vi "High Throughput Streaming - Through Memory (Host).vi"() -> ()   [LabVIEW 2016]
doc: "Example Description:\nStreams data through host memory from a RIO device then back to the RIO device at the specified rate(s).\n\nVI Configuration:\nThis example uses the PXI-7966R as the FPGA target by default. To use this VI with another FPGA target, use the following steps to configure the host VI to use a VI configured for your FPGA target:\n\n1. On the block diagram, right-click the Open FPGA VI Reference (PXI-7966R) VI and select Configure Open FPGA VI Reference.\n2. Browse for a new target by clicking the Browse Project button in the Open VI section.\n3. Select the VI under the target that matches your device. Click OK to select this VI.\n4. Click OK to exit the dialog box and to apply the new selection to the FPGA VI.\n\nRunning the VI:\n1. Select a RIO Resource that corresponds to the FPGA device configured above.\n2. Configure the Requested host Buffer Depth, Read/Write Size, and Requested (M) controls on the Host VI Front Panel.\n3. Click the run arrow to run the VI.\n4. Observe the Status of the Host Buffer as well as the Input and Output DMA FIFOs\n5. Observe the achieved Streaming Throughput.\n6. Click Stop on the Front Panel to stop the example\n\n\nExecution Steps:\nRefer to the block diagram of the Host VI for each example to view the execution steps for that specific example."
uses:
  <vilib>/userdefined/High Color/nirio_resource_hc.ctl
  <vilib>/FPGAPlugInAG/PXIe-7966R/niLvFpga_Open_PXIe-7966R.vi
  <vilib>/rvi/interface/common/dynamic/niFpgaDynamicAddResources.vi
  <vilib>/Utility/error.llb/Error Cluster From Error Code.vi
  <vilib>/rvi/errors/niLvFpgaAdjustHostInterfaceError.vi
  <vilib>/FPGAPlugInAG/Dynamic/niLvFpga_Run_Dynamic.vi
  <vilib>/rvi/interface/common/niFpgaWaitOnOcc.vi
  <vilib>/FPGAPlugInAG/Dynamic/niLvFpga_Close_Dynamic.vi
  <vilib>/rvi/interface/nirviOpenFPGA/nirviOpenFPGA.xnode
  FPGA Bitfiles/HighThroug_PXIe-7966R.lvbitx
  <vilib>/rvi/interface/nirviReadWriteControl/nirviReadWriteControl.xnode
  <vilib>/rvi/interface/nirviMethod/nirviMethod.xnode
  <vilib>/rvi/interface/nirviCloseFPGA/nirviCloseFPGA.xnode
  <vilib>/rvi/interface/Simulation/niFpgaSimulationCallBeginRW.vi
  <vilib>/rvi/errors/niLvFpgaMergeErrorWithErrorCode.vi
  <vilib>/FPGAPlugInAG/Dynamic/niLvFpga_ConfigureFifo_Dynamic.vi
  <vilib>/FPGAPlugInAG/Dynamic/niLvFpga_StartFifo_Dynamic.vi
  <vilib>/FPGAPlugInAG/Dynamic/niLvFpga_AcquireReadRegionFifo_Dynamic.vi
  <vilib>/FPGAPlugInAG/Dynamic/niLvFpga_AcquireWriteRegionFifo_Dynamic.vi
  NiFpgaLv.dll
panel:
  out "error out":errorcluster
  in  "Stop":bool
  out "output.Host Buffer Status":cluster{u32, u32, u32}(slide) caption="Host Output Buffer Status" scale=0.0..67108864.0 scale format="%#.1p"
  out "input.Host Buffer Status":cluster{u32, u32, u32}(slide) caption="Host Input Buffer Status" scale=0.0..67108864.0 scale format="%#.1p"
  out "input.Host Buffer Depth (samples)":u32
  out "output.Host Buffer Depth (samples)":u32
  in  "Read/Write Size (samples)":u32=4194304 step=1048576
  in  "Requested Host Buffer Depth (samples)":u32=67108864 step=1048576
  in  "resource name":T1="Select RIO resource"
  out "output.Ever Timed Out?":bool caption="Overflow"
  in  "output.Reset":bool caption="Reset"
  out "output.FPGA FIFO Status":cluster{u32, u32}(slide) caption="FIFO Status" scale=0.0..65559.0 scale format="%#.1p"
  out "output.Max Throughput":u16 caption="Maximum (M)"
  in  "output.Requested Throughput":u16=1000 caption="Requested (M)" step=5
  out "output.Throughput (B/s)":dbl caption="Actual" format="%#.1p"
  out "input.Ever Timed Out?":bool caption="Overflow"
  in  "input.Reset":bool caption="Reset"
  out "input.FPGA FIFO Status":cluster{u32, u32}(slide) caption="FIFO Status" scale=0.0..65535.0 scale format="%#.1p"
  out "input.Max Throughput":u16 caption="Maximum (M)"
  in  "input.Requested Throughput":u16=1000 caption="Requested (M)" step=5
  out "input.Throughput (B/s)":dbl caption="Actual" format="%#.1p"
  out "Stop...":bool
  # "Configuration"
  # "Host"
  # "Input FPGA"
  # "Throughput (B/s)"
  # "Output FPGA"
  # "Throughput (B/s)"
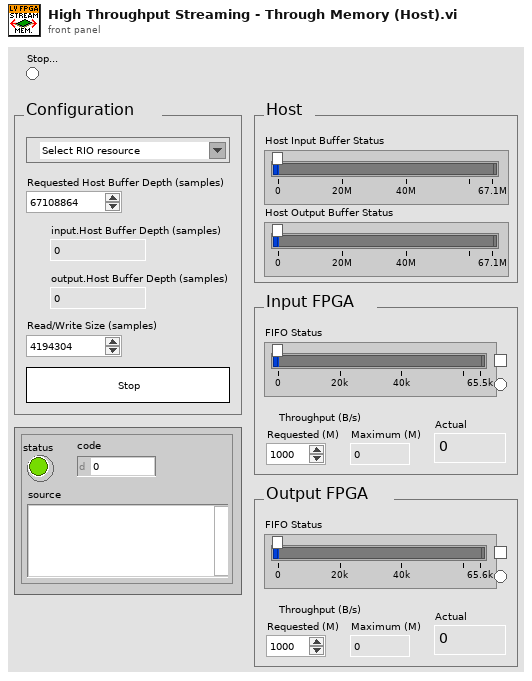
[diagram p1: front panel]
types:
  T1 = typedef "nirio_resource_hc.ctl" = tag
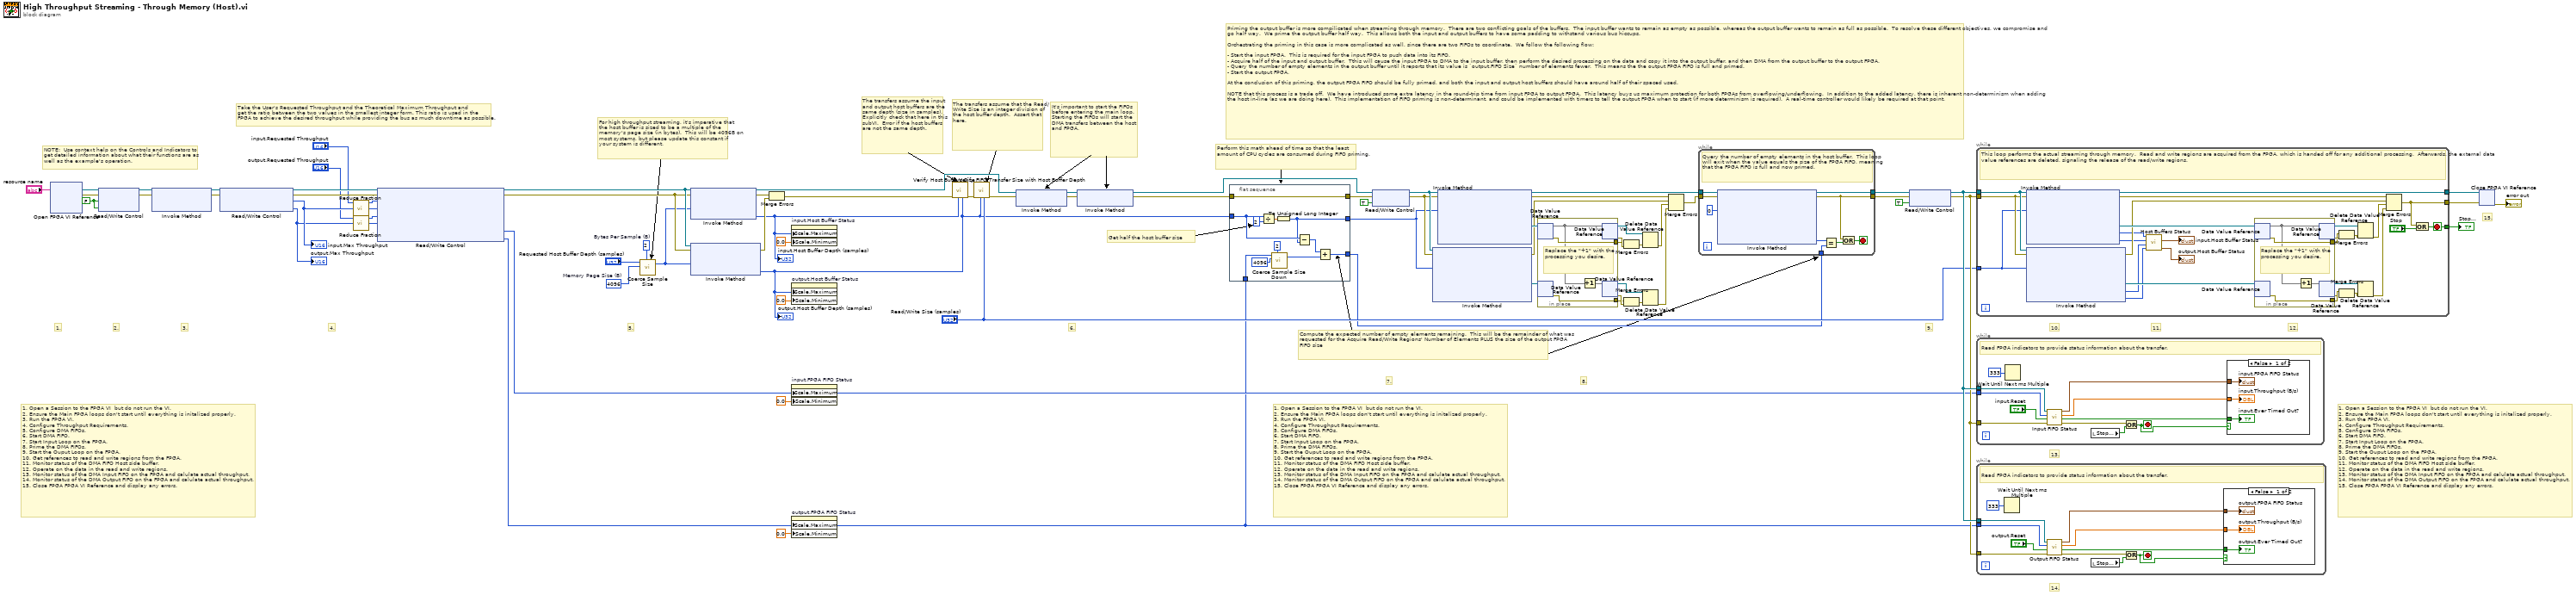
[diagram p0: block diagram]
diagram:
  w60 = u64 4096  # Memory Page Size (B)
  w62 = u64 2  # Bytes Per Sample (B)
  w70 = FALSE ("input.Start")
  # "1. Open a Session to the FPGA VI  but do not run the VI.\n2. Ensure the Main FPGA loops don't start until everything is initalized properly. \n3. Run the FPGA VI.\n4. Configure Throughput Requirements.\n5. Configure DMA FIFOs.\n6. Start DMA FIFO.\n7. Start Input Loop on the FPGA.\n8. Prime the DMA FIFOs.\n9. Start the Ouput Loop on the FPGA.\n10. Get references to read and write regions from the FPGA.\n11. Monitor status of the DMA FIFO Host side buffer.\n12. Operate on the data in the read and write regions. \n13. Monitor status of the DMA Input FIFO on the FPGA and calulate actual throughput.\n14. Monitor status of the DMA Output FIFO on the FPGA and calulate actual throughput.\n15. Close FPGA FPGA VI Reference and display any errors."
  # "1. Open a Session to the FPGA VI  but do not run the VI.\n2. Ensure the Main FPGA loops don't start until everything is initalized properly. \n3. Run the FPGA VI.\n4. Configure Throughput Requirements.\n5. Configure DMA FIFOs.\n6. Start DMA FIFO.\n7. Start Input Loop on the FPGA.\n8. Prime the DMA FIFOs.\n9. Start the Ouput Loop on the FPGA.\n10. Get references to read and write regions from the FPGA.\n11. Monitor status of the DMA FIFO Host side buffer.\n12. Operate on the data in the read and write regions. \n13. Monitor status of the DMA Input FIFO on the FPGA and calulate actual throughput.\n14. Monitor status of the DMA Output FIFO on the FPGA and calulate actual throughput.\n15. Close FPGA FPGA VI Reference and display any errors."
  # "12."
  # "10."
  # "15."
  # "Take the User's Requested Throughput and the Theoretical Maximum Throughput and\nget the ratio between the two values in the smallest integer form. This ratio is used in the \nFPGA to achieve the desired throughput while providing the bus as much downtime as possible."
  # "9."
  # "11."
  # "14."
  # "13."
  # "8."
  # "7."
  # "6."
  # "5."
  # "4."
  # "3."
  # "2."
  # "1. Open a Session to the FPGA VI  but do not run the VI.\n2. Ensure the Main FPGA loops don't start until everything is initalized properly. \n3. Run the FPGA VI.\n4. Configure Throughput Requirements.\n5. Configure DMA FIFOs.\n6. Start DMA FIFO.\n7. Start Input Loop on the FPGA.\n8. Prime the DMA FIFOs.\n9. Start the Ouput Loop on the FPGA.\n10. Get references to read and write regions from the FPGA.\n11. Monitor status of the DMA FIFO Host side buffer.\n12. Operate on the data in the read and write regions. \n13. Monitor status of the DMA Input FIFO on the FPGA and calulate actual throughput.\n14. Monitor status of the DMA Output FIFO on the FPGA and calulate actual throughput.\n15. Close FPGA FPGA VI Reference and display any errors."
  # "1."
  # "NOTE:  Use context help on the Controls and Indicators to \nget detailed information about what their functions are as\nwell as the example's operation."
  # "Compute the expected number of empty elements remaining.  This will be the remainder of what was requested for the Acquire Read/Write Regions' Number of Elements PLUS the size of the output FPGA FIFO size"
  # "Get half the host buffer size"
  # "Perform this math ahead of time so that the least amount of CPU cycles are consumed during FIFO priming."
  # "Priming the output buffer is more compilicated when streaming through memory.  There are two conflicting goals of the buffers.  The input buffer wants to remain as empty as possible, whereas the output buffer wants to remain as full as possible.  To resolve these different objectives, we compromise and go half way.  We prime the output buffer half way.  This allows both the input and output buffers to have some padding to withstand various bus hiccups.\n\nOrchestrating the priming in this case is more complicated as well, since there are two FIFOs to coordinate.  We follow the following flow:\n\n- Start the input FPGA.  This is required for the input FPGA to push data into its FIFO.\n- Acquire half of the input and output buffer.  Tthis will cause the input FPGA to DMA to the input buffer, then perform the desired processing on the data and copy it into the output buffer, and then DMA from the output buffer to the output FPGA.\n- Query the number of empty elements in the output buffer until it reports that its value is `output.FIFO Size` number of elements fewer.  This means the the output FPGA FIFO is full and primed.\n- Start the output FPGA.\n\nAt the conclusion of this priming, the output FPGA FIFO should be fully primed, and both the input and output host buffers should have around half of their spaced used.\n\nNOTE that this process is a trade off.  We have introduced some extra latency in the round-trip time from input FPGA to output FPGA.  This latency buys us maximum protection for both FPGAs from overflowing/underflowing.  In addition to the added latency, there is inherent non-determinism when adding the host in-line (as we are doing here).  This implementation of FIFO priming is non-determinant, and could be implemented with timers to tell the output FPGA when to start (if more determinism is required).  A real-time controller would likely be required at that point."
  # "For high throughput streaming, it's imperative that the host buffer is sized to be a multiple of the memory's page size (in bytes).  This will be 4096B on most systems, but please update this constant if your system is different."
  # "It's important to start the FIFOs before entering the main loop.  Starting the FIFOs will start the DMA transfers between the host and FPGA."
  # "The transfers assume that the Read/Write Size is an integer division of the host buffer depth.  Assert that here."
  # "The transfers assume the input and output host buffers are the same depth (size in samples).  Explicitly check that here in this subVI.  Error if the host buffers are not the same depth."
  n1 = xnode "Open FPGA VI Reference"("resource name"="resource name") -> ("FPGA VI Reference Out"=w72:refnum<k20>, "error out"=w71:errorcluster)  [unwired: 1 in]
  n2 = xnode "Read/Write Control"("FPGA VI Reference In"=w72, "error in"=w71, "input.Start"=w70, "output.Start"=w70) -> ("FPGA VI Reference Out"=w65:refnum<k20>, "error out"=w66:errorcluster)
  n3 = xnode "Invoke Method"("FPGA VI Reference In"=w65, "error in"=w66) -> ("FPGA VI Reference Out"=w42:refnum<k20>, "error out"=w41:errorcluster)  [unwired: 1 in]
  n4 = xnode "Read/Write Control"("FPGA VI Reference In"=w42, "error in"=w41) -> ("FPGA VI Reference Out"=w40:refnum<k20>, "error out"=w39:errorcluster, "input.Max Throughput"=w34:u16, "output.Max Throughput"=w33:u16)
  "input.Max Throughput" <- w34
  "output.Max Throughput" <- w33
  n5 = call "Reduce Fraction.vi"("denominator"=w34, "numerator"="input.Requested Throughput") -> ("reduced denominator"=w38:u16, "reduced numerator"=w35:u16)  [unwired: 2 in]
  n6 = call "Reduce Fraction.vi"("denominator"=w33, "numerator"="output.Requested Throughput") -> ("reduced denominator"=w37:u16, "reduced numerator"=w36:u16)  [unwired: 2 in]
  n7 = xnode "Read/Write Control"("FPGA VI Reference In"=w40, "error in"=w39, "input.Requested Throughput"=w35, "input.Requested Throughput Denominator"=w38, "output.Requested Throughput"=w36, "output.Requested Throughput Denominator"=w37) -> ("FPGA VI Reference Out"=w58:refnum<k20>, "error out"=w57:errorcluster, "input.FIFO Size"=w43:u32, "output.FIFO Size"=w8:u32)
  n8 = call "Coerce Sample Size.vi"("Bytes Per Sample (B)"=w62, "Coerce To (B)"=w60, "Size (samples)"="Requested Host Buffer Depth (samples)") -> ("Coerced Size (samples)"=w56:u64)  [unwired: 4 in]
  n9 = xnode "Invoke Method"("FPGA VI Reference In"=w58, "error in"=w57, "Requested Depth"=w56) -> ("FPGA VI Reference Out"=w49:refnum<k20>, "error out"=w54:errorcluster, "Actual Depth"=w1:u32)
  "input.Host Buffer Depth (samples)" <- w1
  n10 = xnode "Invoke Method"("FPGA VI Reference In"=w58, "error in"=w57, "Requested Depth"=w56) -> ("error out"=w53:errorcluster, "Actual Depth"=w2:u32)  [unwired: 1 out]
  "output.Host Buffer Depth (samples)" <- w2
  n11 = Merge Errors(w54, w53) -> (w52:errorcluster)
  n12 = property on="input.Host Buffer Status" class="Slide (strict)"("Scale.Maximum"=w1, "Scale.Minimum"=0.0 ("Scale.Range:Minimum")) -> ()  [unwired: 2 in, 2 out]
  n13 = property on="output.Host Buffer Status" class="Slide (strict)"("Scale.Maximum"=w2, "Scale.Minimum"=0.0 ("Scale.Range:Minimum")) -> ()  [unwired: 2 in, 2 out]
  n14 = property on="input.FPGA FIFO Status" class="Slide (strict)"("Scale.Maximum"=w43, "Scale.Minimum"=0.0 ("Scale.Range:Minimum")) -> ()  [unwired: 2 in, 2 out]
  n15 = property on="output.FPGA FIFO Status" class="Slide (strict)"("Scale.Maximum"=w8, "Scale.Minimum"=0.0 ("Scale.Range:Minimum")) -> ()  [unwired: 2 in, 2 out]
  n16 = call "Verify Host Buffers Size.vi"("output.Host Buffer Size"=w2, "input.Host Buffer Size"=w1, "error in"=w52) -> ("error out"=w51:errorcluster)  [unwired: 8 in]
  n17 = call "Verify FIFO Transfer Size with Host Buffer Depth.vi"("Read/Write Size (samples)"="Read/Write Size (samples)", "Host Buffer Depth (samples)"=w2, "error in"=w51) -> ("error out"=w48:errorcluster)  [unwired: 8 in]
  n18 = xnode "Invoke Method"("FPGA VI Reference In"=w49, "error in"=w48) -> ("FPGA VI Reference Out"=w46:refnum<k20>, "error out"=w47:errorcluster)
  n19 = xnode "Invoke Method"("FPGA VI Reference In"=w46, "error in"=w47) -> ("FPGA VI Reference Out"=w4:refnum<k20>, "error out"=w6:errorcluster)
  n20 = flat-sequence {
    tunnel: w8 -> [w83]
    tunnel: w2 -> [w82]
    tunnel: [w78] -> w7
    tunnel: w6 -> [w77]
    tunnel: [w77] -> w5
    tunnel: [w75] -> w3
    frame #0 {
      n21 = Divide(x=w82, y=u32 2) -> (x/y=w79:dbl)
      n22 = call "Coerce Sample Size Down.vi"("Bytes Per Sample (B)"=u64 2, "Coerce To (B)"=u64 4096, "Size (samples)"=w83) -> ("Coerced Size (samples)"=w80:u64)  [unwired: 4 in]
      n23 = To Unsigned Long Integer(number=w79) -> (unsigned 32bit integer=w78:u32)
      n24 = Subtract(x=w82, y=w78) -> (x-y=w81:u32)
      n25 = Add(x=w81, y=w80) -> (x+y=w75:u64)
    }
  }
  n26 = xnode "Read/Write Control"("FPGA VI Reference In"=w4, "error in"=w5, "input.Start"=TRUE) -> ("FPGA VI Reference Out"=w29:refnum<k20>, "error out"=w28:errorcluster)
  n27 = xnode "Invoke Method"("FPGA VI Reference In"=w29, "error in"=w28, "Number of Elements"=w7) -> ("error out"=w14:errorcluster, "Write Region Reference"=w26:refnum<data-value>)  [unwired: 1 in, 3 out]
  n28 = xnode "Invoke Method"("FPGA VI Reference In"=w29, "error in"=w28, "Number of Elements"=w7) -> ("FPGA VI Reference Out"=w10:refnum<k20>, "error out"=w25:errorcluster, "Read Region Reference"=w27:refnum<data-value>)  [unwired: 1 in, 2 out]
  n29 = in-place {
    in-place-border: [w89] -> w19
    in-place-border: [w88] -> w17
    # "Replace the \"+1\" with the processing you desire."
    # "Insert additional processing here"
    n30 = in-place-dvr #1(w27) -> (w87:i16[], w88:errorcluster)
    n31 = in-place-dvr #2(w26) -> (w89:errorcluster)  [unwired: 1 out]
    n32 = Increment(x=w87) -> (x+1=w86:i16[])
    n33 = in-place-dvr #1(w87) -> (w22:refnum<data-value>, w18:errorcluster)
    n34 = in-place-dvr #2(w86) -> (w21:refnum<data-value>, w20:errorcluster)
  }
  n35 = Merge Errors(w17, w18) -> (w24:errorcluster)
  n36 = Merge Errors(w19, w20) -> (w23:errorcluster)
  n37 = Delete Data Value Reference(data value reference=w22, error in=w24) -> (error out=w15:errorcluster)  [unwired: 1 out]
  n38 = Delete Data Value Reference(data value reference=w21, error in=w23) -> (error out=w16:errorcluster)  [unwired: 1 out]
  n39 = Merge Errors(w25, w14, w15, w16) -> (w9:errorcluster)
  n40 = while {
    tunnel: w9 -> [w98]
    tunnel: [w95] -> w12
    tunnel: w10 -> [w97]
    tunnel: w3 -> [w93]
    tunnel: [w90] -> w11
    stop <- w96 stop-if-true
    # "Query the number of empty elements in the host buffer.  This loop will exit when the value equals the size of the FPGA FIFO, meaning that the FPGA FIFO is full and now primed."
    n41 = xnode "Invoke Method"("FPGA VI Reference In"=w97, "error in"=w98, "Number of Elements"=u32 0) -> ("FPGA VI Reference Out"=w90:refnum<k20>, "error out"=w95:errorcluster, "Empty Elements Remaining"=w91:u32)  [unwired: 1 in, 2 out]
    n42 = Equal?(x=w91, y=w93) -> (x = y?=w94:bool)
    n43 = Or(x=w95, y=w94) -> (x .or. y?=w96:bool)
  }
  n44 = xnode "Read/Write Control"("FPGA VI Reference In"=w11, "error in"=w12, "output.Start"=TRUE ("Start")) -> ("FPGA VI Reference Out"=w64:refnum<k20>, "error out"=w63:errorcluster)
  n45 = while {
    tunnel: w64 -> [w125]
    tunnel: w63 -> [w124]
    tunnel: "Read/Write Size (samples)" -> [w107]
    tunnel: [w119] -> w69
    tunnel: [w118] -> w67
    tunnel: [w116] -> w68
    stop <- w116 stop-if-true
    # "This loop performs the actual streaming through memory.  Read and write regions are acquired from the FPGA, which is handed off for any additional processing.  Afterwards, the external data value references are deleted, signaling the release of the read/write regions."
    n46 = xnode "Invoke Method"("FPGA VI Reference In"=w125, "error in"=w124, "Number of Elements"=w107) -> ("FPGA VI Reference Out"=w119:refnum<k20>, "error out"=w106:errorcluster, "Read Region Reference"=w123:refnum<data-value>, "Elements In Region"=w99:u32, "Elements Remaining"=w102:u32)  [unwired: 1 in]
    n47 = xnode "Invoke Method"("FPGA VI Reference In"=w125, "error in"=w124, "Number of Elements"=w107) -> ("error out"=w105:errorcluster, "Write Region Reference"=w122:refnum<data-value>, "Elements In Region"=w104:u32, "Empty Elements Remaining"=w103:u32)  [unwired: 1 in, 1 out]
    n48 = call "Host Buffers Status.vi"("output.Empty Elements Remaining"=w103, "output.Elements In Region"=w104, "input.Elements Remaining"=w102, "input.Elements In Region"=w99) -> ("output.Host Buffer Status"=→"output.Host Buffer Status":cluster{u32, u32, u32}, "input.Host Buffer Status"=→"input.Host Buffer Status":cluster{u32, u32, u32})  [unwired: 4 in, 2 out]
    n49 = in-place {
      in-place-border: [w129] -> w111
      in-place-border: [w128] -> w108
      # "Replace the \"+1\" with the processing you desire."
      # "Insert additional processing here"
      n50 = in-place-dvr #3(w123) -> (w127:i16[], w128:errorcluster)
      n51 = in-place-dvr #4(w122) -> (w129:errorcluster)  [unwired: 1 out]
      n52 = Increment(x=w127) -> (x+1=w126:i16[])
      n53 = in-place-dvr #3(w127) -> (w115:refnum<data-value>, w109:errorcluster)
      n54 = in-place-dvr #4(w126) -> (w114:refnum<data-value>, w110:errorcluster)
    }
    n55 = Merge Errors(w108, w109) -> (w112:errorcluster)
    n56 = Merge Errors(w111, w110) -> (w113:errorcluster)
    n57 = Delete Data Value Reference(data value reference=w115, error in=w112) -> (error out=w121:errorcluster)  [unwired: 1 out]
    n58 = Delete Data Value Reference(data value reference=w114, error in=w113) -> (error out=w120:errorcluster)  [unwired: 1 out]
    n59 = Merge Errors(w106, w105, w121, w120) -> (w118:errorcluster)
    n60 = Compound Arithmetic op=OR(w118, "Stop") -> (w116:bool)
  }
  "Stop..." <- w68
  n61 = while {
    tunnel: w63 -> [w138]
    tunnel: w43 -> [w136]
    tunnel: w64 -> [w135]
    stop <- w130 stop-if-true
    # "Read FPGA indicators to provide status information about the transfer."
    n62 = Wait Until Next ms Multiple(millisecond multiple=u32 333) -> ()  [unwired: 1 out]
    n63 = call "Input FIFO Status.vi"("error in"=w138, "input.Reset"="input.Reset", "input.FIFO Size"=w136, "FPGA VI Reference"=w135) -> ("error out"=w134:errorcluster, "input.Ever Timed Out?"=w133:bool, "input.Throughput (B/s)"=w132:dbl, "input.FPGA FIFO Status"=w131:cluster{u32, u32})  [unwired: 3 in]
    n64 = local read "Stop..."() -> (w139:bool)
    n65 = Or(x=w134, y=w139) -> (x .or. y?=w130:bool)
    n66 = case shown="False" w130 {
      tunnel: w133 -> [w143 _]
      tunnel: w132 -> [w142 _]
      tunnel: w131 -> [w141 _]
      frame False {
        "input.Throughput (B/s)" <- w142
        "input.Ever Timed Out?" <- w143
        "input.FPGA FIFO Status" <- w141
      }
      frame True {
      }
    }
  }
  n67 = while {
    tunnel: w64 -> [w145]
    tunnel: w63 -> [w153]
    tunnel: w8 -> [w151]
    stop <- w144 stop-if-true
    # "Read FPGA indicators to provide status information about the transfer."
    n68 = Wait Until Next ms Multiple(millisecond multiple=u32 333) -> ()  [unwired: 1 out]
    n69 = call "Output FIFO Status.vi"("error in"=w153, "output.Reset"="output.Reset", "output.FIFO Size"=w151, "FPGA VI Reference"=w145) -> ("error out"=w150:errorcluster, "output.Ever Timed Out?"=w148:bool, "output.Throughput (B/s)"=w147:dbl, "output.FPGA FIFO Status"=w146:cluster{u32, u32})  [unwired: 4 in]
    n70 = local read "Stop..."() -> (w149:bool)
    n71 = Or(x=w150, y=w149) -> (x .or. y?=w144:bool)
    n72 = case shown="False" w144 {
      tunnel: w148 -> [w157 _]
      tunnel: w147 -> [w156 _]
      tunnel: w146 -> [w155 _]
      frame False {
        "output.Throughput (B/s)" <- w156
        "output.Ever Timed Out?" <- w157
        "output.FPGA FIFO Status" <- w155
      }
      frame True {
      }
    }
  }
  n73 = xnode "Close FPGA VI Reference"("FPGA VI Reference In"=w69, "error in"=w67) -> ("error out"=→"error out":errorcluster)
